vi "app -- vew -- meta PID.vi"() -> ()   [LabVIEW 2015]
uses:
  ctl -- name dispatcher -- action.ctl
  tale of three indices.vi
  linear interpolation - real.vi
  line -- complex.vi
  Q -- check range -- i -- integer.vi
  command stack.vi
  tale of three indices -- check state.vi
  Q - not nan -- integer.vi
panel:
  in  "N":i32(slide)=1000 min=-506096563 max=2129711151 step=1 scale=0.01..1000.0
  in  "T max":dbl(slide)=3081.6920476849527 min=-506096563.00000006 max=2129711151.0 step=0.010000000000000002 scale=0.01..10000.0 scale format="%#3_3f"
  in  "T min":dbl(slide)=30.856999999959953 min=-506096563.00000006 max=2129711151.0 step=0.010000000000000002 scale=0.01..1000.0 scale format="%#3_3f"
  in  "divide T by":i32=1
  in  "ctl name dispatch":T1=enum."set temperature "
  out "Plot: phase space - slope vs var":cluster{dbl[], dbl[]}[](graph)
  out "Plot: slope":cluster{dbl[], dbl[]}[](graph)
  out "ok":bool=TRUE
  in  "sweep folder path":path=path "D:/Technique/RUS/CeCu2Si2/A116/2_cooling"
  out "Plot: var":cluster{dbl[], dbl[]}[](graph)=[{[0.0, 200.0, 600.0, 800.0, 1200.0], [88.769, 60.0, 30.0, 20.0, 5.0]}, {array[1000 elements], array[1000 elements]}]
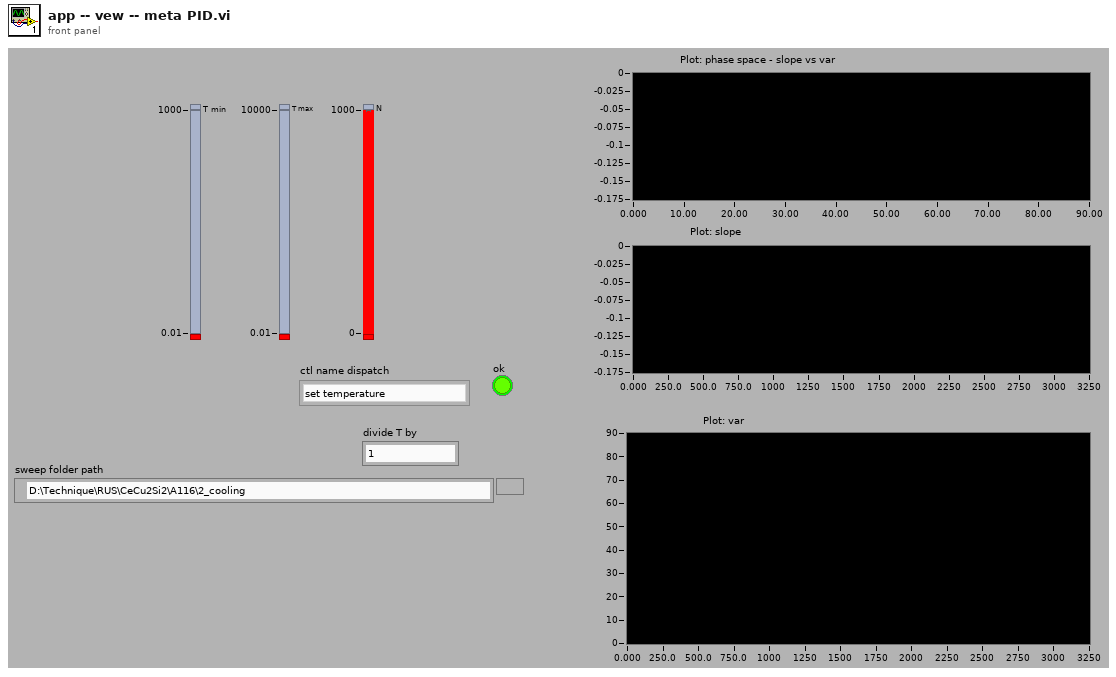
[diagram p1: front panel]
types:
  T1 = typedef "ctl -- name dispatcher -- action.ctl" = enum16{"peak frequency", "peak frequency DUMP", "peak gamma DUMP", "peak gamma", "peak frequency TEST", "peak gamma TEST", "ultrasonic power", "time in gamma", "set temperature ", "set temperature timer", "peak default gamma", "last scan file", "peak freq gamma TEST", "peak NAMES", "errors", "P_I_D", "P", "I", "D", "power vs time", "power vs time TIMER", "void", "power log", "set temperature - SINE", "itc ltc log", "peak - time in gamma"}
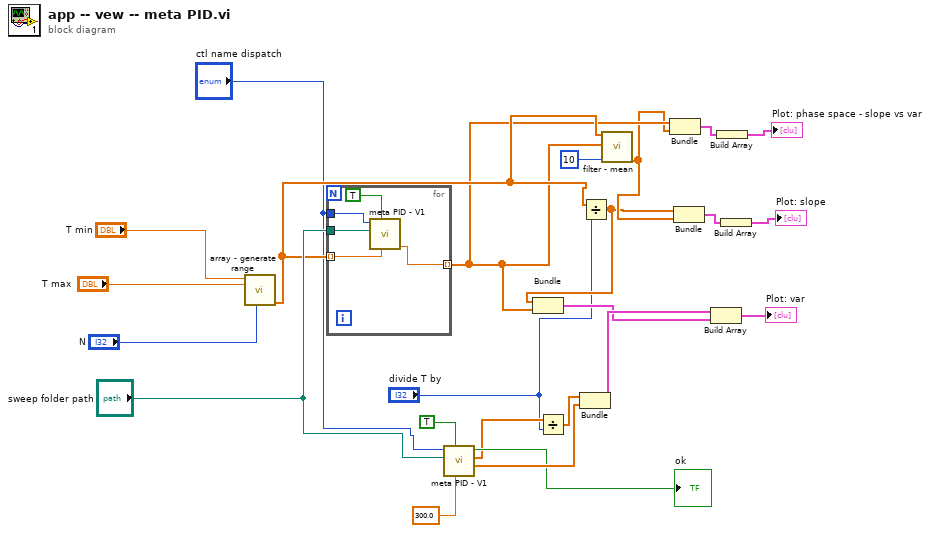
[diagram p0: block diagram]
diagram:
  n1 = call "array - generate range.vi"("N"="N", "freq max"="T max", "freq min"="T min") -> ("Array"=w13:dbl[])  [unwired: 7 in, 1 out]
  n2 = for {
    tunnel: w13 -> [w28] mode=indexing
    tunnel: [w27] -> w10 mode=indexing
    tunnel: "sweep folder path" -> [w29]
    tunnel: "ctl name dispatch" -> [w25]
    n3 = call "meta PID - V1.vi"("input parameter"=w28, "control?"=TRUE ("control power PID?"), "sweep folder path"=w29, "ctl name dispatch"=w25) -> ("bezier output"=w27:dbl)  [unwired: 4 in, 3 out]
  }
  n4 = call "meta PID - V1.vi"("input parameter"=300.0 ("nonzero temperature"), "control?"=TRUE ("control power PID?"), "sweep folder path"="sweep folder path", "ctl name dispatch"="ctl name dispatch") -> ("frequencies"=w21:dbl[], "temperatures"=w7:dbl[], "ok"=→"ok":bool)  [unwired: 4 in, 1 out]
  n5 = Divide(x=w7, y="divide T by") -> (x/y=w5:dbl[])
  n6 = Bundle(w5, "frequencies"=w21) -> (w24:cluster{dbl[], "frequencies":dbl[]})  [unwired: 1 in]
  n7 = Divide(x=w13, y="divide T by") -> (x/y=w8:dbl[])
  n8 = Bundle(w8, w10) -> (w23:cluster{dbl[], dbl[]})  [unwired: 1 in]
  n9 = call "filter - mean.vi"("omega  in"=w13, "z in"=w10, "window"=10) -> ("slope"=w9:dbl[])  [unwired: 13 in, 3 out]
  n10 = Bundle(w10, "slope"=w9) -> (w12:cluster{dbl[], "slope":dbl[]})  [unwired: 1 in]
  n11 = Bundle(w8, "slope"=w9) -> (w16:cluster{dbl[], "slope":dbl[]})  [unwired: 1 in]
  n12 = Build Array(w24, w23) -> (→"Plot: var":cluster{dbl[], "frequencies":dbl[]}[])
  n13 = Build Array(w12) -> (→"Plot: phase space - slope vs var":cluster{dbl[], "slope":dbl[]}[])
  n14 = Build Array(w16) -> (→"Plot: slope":cluster{dbl[], "slope":dbl[]}[])
